vi "Copy Template Files.vi"(8 "error in (no error)":errorcluster, 10 "Server Library (Library Item) in":refnum<vi>, 11 "Template Library (Library Item) in":refnum<vi>) -> (0 "error out":errorcluster, 2 "Server Library (Library Item) out":refnum<vi>, 3 "Template Library (Library Item) out":refnum<vi>)   [LabVIEW 2019, in "gRPC Template Creation Utility.lvlib"]
uses:
  gRPC Template Creation Utility.lvlib
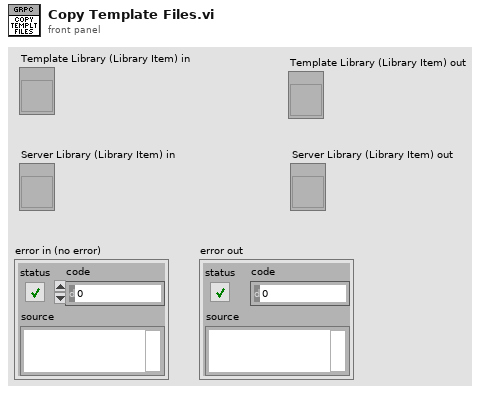
[diagram p1: front panel]
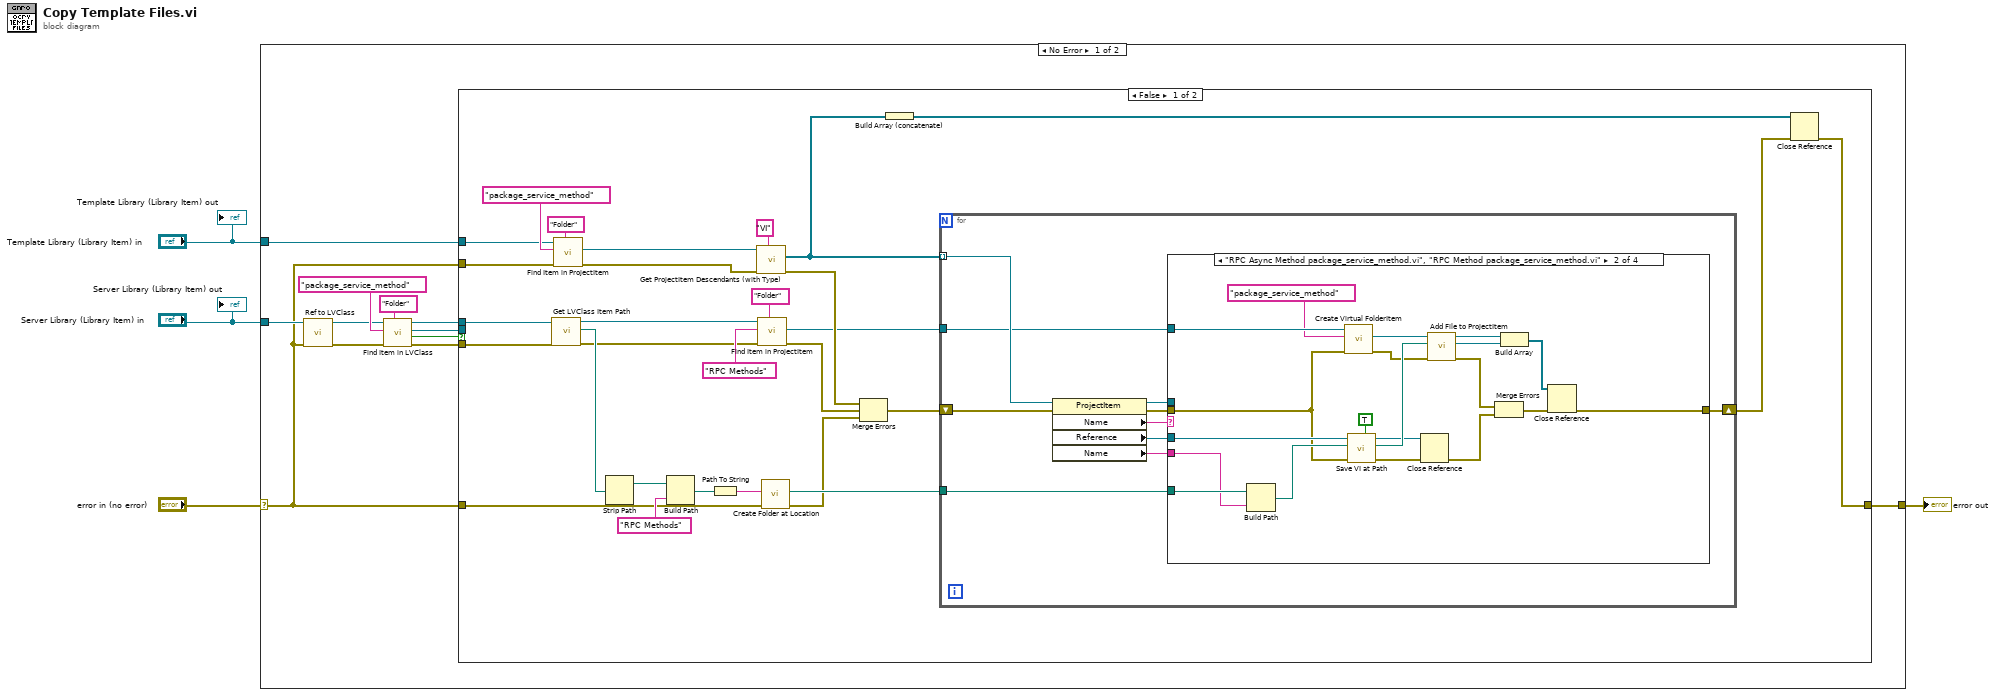
[diagram p0: block diagram]
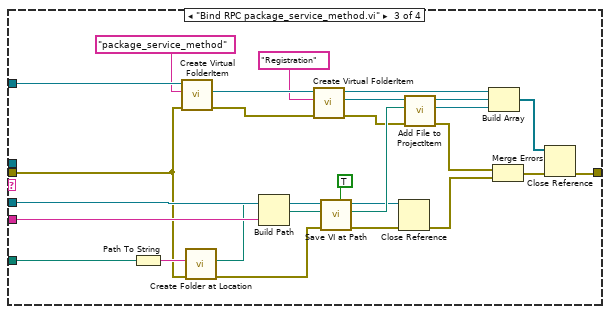
[diagram p3: hidden frame]
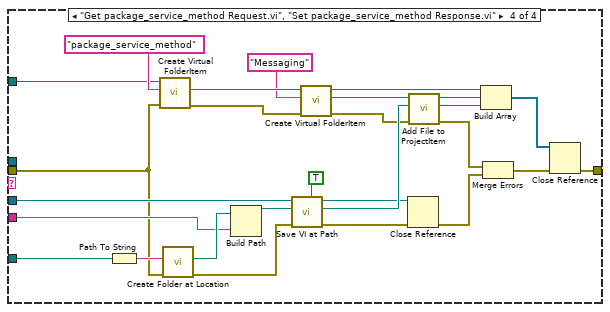
[diagram p4: hidden frame]
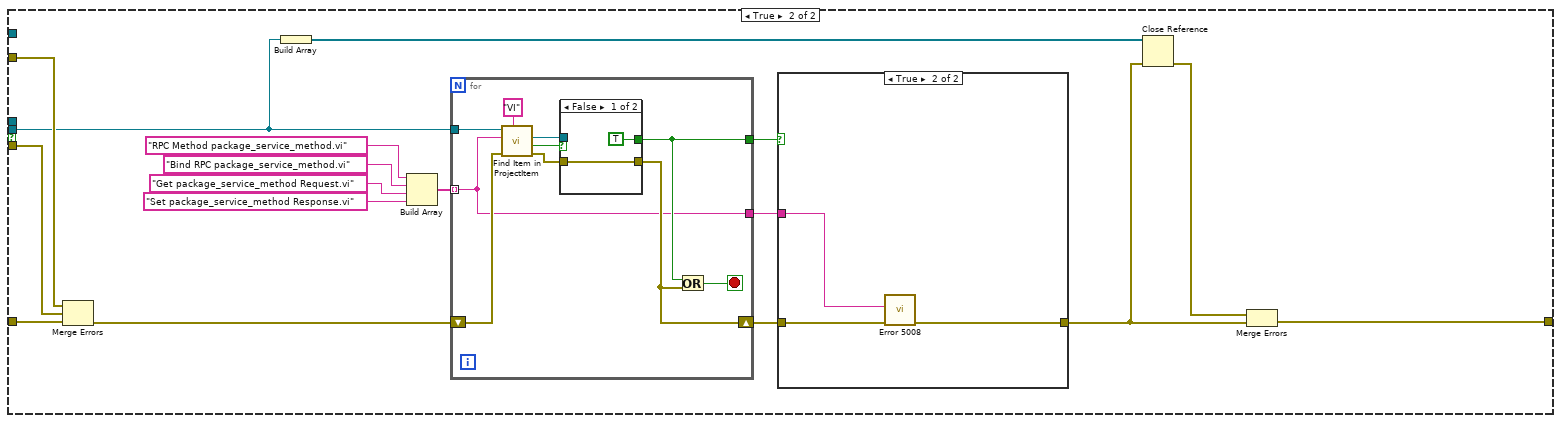
[diagram p5: hidden frame]
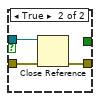
[diagram p7: hidden frame]
diagram:
  n1 = case shown="No Error" "error in (no error)" {
    selector: "error in (no error)" -> [w6 w166]
    tunnel: "Template Library (Library Item) in" -> [w9 _]
    tunnel: "Server Library (Library Item) in" -> [w8 _]
    tunnel: [w16 w166] -> w1
    frame No Error {
      n2 = call "Ref to LVClass.vi"("error in (no error)"=w6, "ProjectItem in"=w8) -> ("error out"=w5:errorcluster, "LVClassLibrary out"=w7:refnum<vi>)  [unwired: 8 in]
      n3 = call "Find Item in LVClass.vi"("Item Type"="Folder", "error in (no error)"=w5, "Item Name"="package_service_method" ("Name"), "Class Item in"=w7) -> ("error out"=w11:errorcluster, "Found?"=w13:bool, "Project Item (Class Item)"=w10:refnum<vi>, "Class Item out"=w12:refnum<vi>)  [unwired: 4 in]
      n4 = case shown="False" w13 {
        tunnel: w9 -> [w43 _]
        tunnel: w6 -> [w33 w146]
        tunnel: w6 -> [w32 w144]
        tunnel: [w22 w132] -> w16
        tunnel: w11 -> [w17 w145]
        tunnel: w12 -> [w18 _]
        tunnel: w10 -> [_ w142]
        frame False {
          n5 = call "Get LVClass Item Path.vi"("error in (no error)"=w17, "LVClassLibrary in"=w18) -> ("error out"=w19:errorcluster, "Path"=w21:path, "LVClassLibrary out"=w20:refnum<vi>)  [unwired: 7 in]
          n6 = call "Find Item in ProjectItem.vi"("Item Type"="Folder", "error in (no error)"=w32, "Name"="package_service_method", "ProjectItem in"=w43) -> ("error out"=w31:errorcluster, "Item Refnum out"=w42:refnum<vi>)  [unwired: 4 in, 2 out]
          n7 = Strip Path(path=w21) -> (stripped path=w40:path)  [unwired: 1 out]
          n8 = Build Path(base path=w40, name or relative path="RPC Methods") -> (appended path=w38:path)
          n9 = Path To String(path=w38) -> (string=w37:string)
          n10 = call "Get ProjectItem Descendants (with Type).vi"("Type"="VI", "error in (no error)"=w31, "ProjectItem in"=w42) -> ("error out"=w29:errorcluster, "All Descendents"=w26:refnum<vi>[])  [unwired: 6 in, 1 out]
          n11 = call "Find Item in ProjectItem.vi"("Item Type"="Folder", "error in (no error)"=w19, "Name"="RPC Methods", "ProjectItem in"=w20) -> ("error out"=w28:errorcluster, "Item Refnum out"=w25:refnum<vi>)  [unwired: 4 in, 2 out]
          n12 = call "Create Folder at Location.vi"("Error In"=w33, "Path"=w37) -> ("Error Out"=w30:errorcluster, "Full path out"=w36:path)  [unwired: 7 in, 1 out]
          n13 = Merge Errors(w29, w28, w30) -> (w27:errorcluster)
          n14 = Build Array (concatenate)(w26) -> (w24:refnum<vi>[])
          n15 = for {
            tunnel: w26 -> [w55] mode=indexing
            tunnel: w36 -> [w52]
            tunnel: w25 -> [w50]
            shift-right: [w46] -> w23
            shift-left: w27 -> [w48]
            n16 = property class="ProjectItem"(reference=w55, error in=w48) -> (reference out=w53:refnum<vi>, error out=w47:errorcluster, "Name"=w54:string, "Reference"=w49:refnum<vi>, "Name"=w51:string)
            n17 = case shown="\"RPC Async Method package_service_method.vi\", \"RPC Method package_service_method.vi\"" w54 {
              tunnel: w53 -> [_ _ _ _]
              tunnel: w52 -> [_ w76 w101 w129]
              tunnel: w51 -> [_ w75 w103 w126]
              tunnel: w50 -> [_ w74 w95 w121]
              tunnel: w49 -> [_ w70 w100 w124]
              tunnel: w47 -> [w56 w67 w91 w117]
              tunnel: [w56 w60 w80 w107] -> w46
              frame "None", Default {
              }
              frame "RPC Async Method package_service_method.vi", "RPC Method package_service_method.vi" {
                n18 = Build Path(base path=w76, name or relative path=w75) -> (appended path=w69:path)
                n19 = call "Create Virtual FolderItem.vi"("error in (no error)"=w67, "Folder Name"="package_service_method", "ProjectItem in"=w74) -> ("error out"=w66:errorcluster, "FolderItem reference out"=w72:refnum<vi>)  [unwired: 5 in, 2 out]
                n20 = call "Save VI at Path.vi"("Save a Copy (F)"=TRUE, "error in (no error)"=w67, "Path"=w69, "VI in"=w70) -> ("error out"=w59:errorcluster, "Path to saved File"=w68:path, "VI out"=w58:refnum<vi>)  [unwired: 5 in]
                n21 = Close Reference(reference=w58, error in (no error)=w59) -> (error out=w57:errorcluster)
                n22 = call "Add File to ProjectItem.vi"("error in (no error)"=w66, "File Path"=w68, "ProjectItem in"=w72) -> ("error out"=w65:errorcluster, "Added File ref"=w63:refnum<vi>, "ProjectItem out"=w64:refnum<vi>)  [unwired: 6 in]
                n23 = Merge Errors(w65, w57) -> (w62:errorcluster)
                n24 = Build Array(w64, w63) -> (w61:refnum<vi>[])
                n25 = Close Reference(reference=w61, error in (no error)=w62) -> (error out=w60:errorcluster)
              }
              frame "Bind RPC package_service_method.vi" {
                n26 = Path To String(path=w101) -> (string=w102:string)
                n27 = call "Create Virtual FolderItem.vi"("error in (no error)"=w91, "Folder Name"="package_service_method", "ProjectItem in"=w95) -> ("error out"=w90:errorcluster, "FolderItem reference out"=w97:refnum<vi>)  [unwired: 5 in, 2 out]
                n28 = call "Create Folder at Location.vi"("Error In"=w91, "Path"=w102) -> ("Error Out"=w88:errorcluster, "Full path out"=w87:path)  [unwired: 7 in, 1 out]
                n29 = Build Path(base path=w87, name or relative path=w103) -> (appended path=w98:path)
                n30 = call "Create Virtual FolderItem.vi"("error in (no error)"=w90, "Folder Name"="Registration", "ProjectItem in"=w97) -> ("error out"=w89:errorcluster, "FolderItem reference out"=w92:refnum<vi>, "ProjectItem out"=w84:refnum<vi>)  [unwired: 5 in, 1 out]
                n31 = call "Save VI at Path.vi"("Save a Copy (F)"=TRUE, "error in (no error)"=w88, "Path"=w98, "VI in"=w100) -> ("error out"=w79:errorcluster, "Path to saved File"=w93:path, "VI out"=w78:refnum<vi>)  [unwired: 5 in]
                n32 = Close Reference(reference=w78, error in (no error)=w79) -> (error out=w77:errorcluster)
                n33 = call "Add File to ProjectItem.vi"("error in (no error)"=w89, "File Path"=w93, "ProjectItem in"=w92) -> ("error out"=w86:errorcluster, "Added File ref"=w82:refnum<vi>, "ProjectItem out"=w83:refnum<vi>)  [unwired: 6 in]
                n34 = Build Array(w84, w83, w82) -> (w81:refnum<vi>[])
                n35 = Merge Errors(w86, w77) -> (w85:errorcluster)
                n36 = Close Reference(reference=w81, error in (no error)=w85) -> (error out=w80:errorcluster)
              }
              frame "Get package_service_method Request.vi", "Set package_service_method Response.vi" {
                n37 = Path To String(path=w129) -> (string=w128:string)
                n38 = call "Create Virtual FolderItem.vi"("error in (no error)"=w117, "Folder Name"="package_service_method", "ProjectItem in"=w121) -> ("error out"=w115:errorcluster, "FolderItem reference out"=w120:refnum<vi>)  [unwired: 5 in, 2 out]
                n39 = call "Create Folder at Location.vi"("Error In"=w117, "Path"=w128) -> ("Error Out"=w116:errorcluster, "Full path out"=w127:path)  [unwired: 7 in, 1 out]
                n40 = Build Path(base path=w127, name or relative path=w126) -> (appended path=w123:path)
                n41 = call "Save VI at Path.vi"("Save a Copy (F)"=TRUE, "error in (no error)"=w116, "Path"=w123, "VI in"=w124) -> ("error out"=w106:errorcluster, "Path to saved File"=w118:path, "VI out"=w105:refnum<vi>)  [unwired: 5 in]
                n42 = call "Create Virtual FolderItem.vi"("error in (no error)"=w115, "Folder Name"="Messaging", "ProjectItem in"=w120) -> ("error out"=w114:errorcluster, "FolderItem reference out"=w111:refnum<vi>, "ProjectItem out"=w112:refnum<vi>)  [unwired: 5 in, 1 out]
                n43 = Close Reference(reference=w105, error in (no error)=w106) -> (error out=w104:errorcluster)
                n44 = call "Add File to ProjectItem.vi"("error in (no error)"=w114, "File Path"=w118, "ProjectItem in"=w111) -> ("error out"=w113:errorcluster, "Added File ref"=w110:refnum<vi>)  [unwired: 6 in, 1 out]
                n45 = Build Array(w112, w111, w110) -> (w108:refnum<vi>[])
                n46 = Merge Errors(w113, w104) -> (w109:errorcluster)
                n47 = Close Reference(reference=w108, error in (no error)=w109) -> (error out=w107:errorcluster)
              }
            }
          }
          n48 = Close Reference(reference=w24, error in (no error)=w23) -> (error out=w22:errorcluster)
        }
        frame True {
          n49 = Merge Errors(w144, w145, w146) -> (w136:errorcluster)
          n50 = Build Array(w142) -> (w143:refnum<vi>[])
          n51 = Build Array("RPC Method package_service_method.vi" ("Name"), "Bind RPC package_service_method.vi" ("element"), "Get package_service_method Request.vi" ("element"), "Set package_service_method Response.vi" ("element")) -> (w137:string[])
          n52 = for {
            tunnel: w142 -> [w160]
            tunnel: w137 -> [w151] mode=indexing
            shift-right: [w153] -> w135
            shift-left: w136 -> [w156]
            tunnel: [w152] -> w134
            tunnel: [w151] -> w133
            stop <- w154 stop-if-true
            n53 = call "Find Item in ProjectItem.vi"("Item Type"="VI", "error in (no error)"=w156, "Name"=w151, "ProjectItem in"=w160) -> ("error out"=w155:errorcluster, "Found ?"=w158:bool, "Item Refnum out"=w157:refnum<vi>)  [unwired: 4 in, 1 out]
            n54 = case shown="False" w158 {
              tunnel: w157 -> [_ w165]
              tunnel: w155 -> [w162 w164]
              tunnel: [w162 w163] -> w153
              tunnel: [TRUE _] -> w152
              frame False {
              }
              frame True {
                n55 = Close Reference(reference=w165, error in (no error)=w164) -> (error out=w163:errorcluster)
              }
            }
            n56 = Or(x=w152, y=w153) -> (x .or. y?=w154:bool)
          }
          n57 = case shown="True" w134 {
            tunnel: w135 -> [w147 w150]
            tunnel: w133 -> [_ w149]
            tunnel: [w147 w148] -> w130
            frame False {
            }
            frame True {
              n58 = call "Error 5008.vi"("error in (no error)"=w150, "File Name"=w149) -> ("error out"=w148:errorcluster)  [unwired: 9 in]
            }
          }
          n59 = Close Reference(reference=w143, error in (no error)=w130) -> (error out=w131:errorcluster)
          n60 = Merge Errors(w131, w130) -> (w132:errorcluster)
        }
      }
    }
    frame Error {
    }
  }
  "error out" <- w1
  "Template Library (Library Item) out" <- "Template Library (Library Item) in"
  "Server Library (Library Item) out" <- "Server Library (Library Item) in"
